vi "Read.vi"(0 "QCS in":refnum<class "QCS.lvclass">, 5 "error in (no error)":errorcluster, 6 "Force error check\nat low range":bool) -> (14 "QCS out":refnum<class "QCS.lvclass">, 15 "I0":T1 {"Current" min=0.0}, 16 "I1":T1 {"Current" min=0.0}, 17 "I2":T1 {"Current" min=0.0}, 18 "I3":T1 {"Current" min=0.0}, 19 "error out":errorcluster)   [LabVIEW 2013, in "QCS.lvclass"]
uses:
  Lib.llb/QCS.lvclass
  Lib.llb/CS Data.ctl
  Lib.llb/CS.lvclass
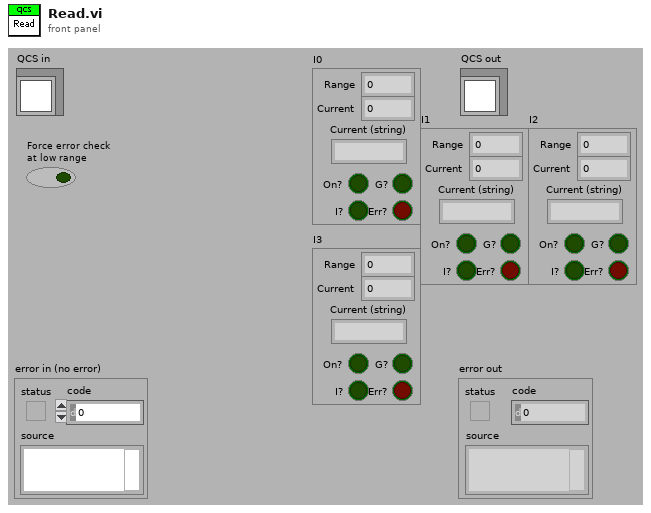
[diagram p1: front panel]
types:
  T1 = typedef "CS Data.ctl" = cluster{"Range":u8, "Current":dbl, "Current (string)":string, "On?":bool, "G?":bool, "I?":bool, "Err?":bool}
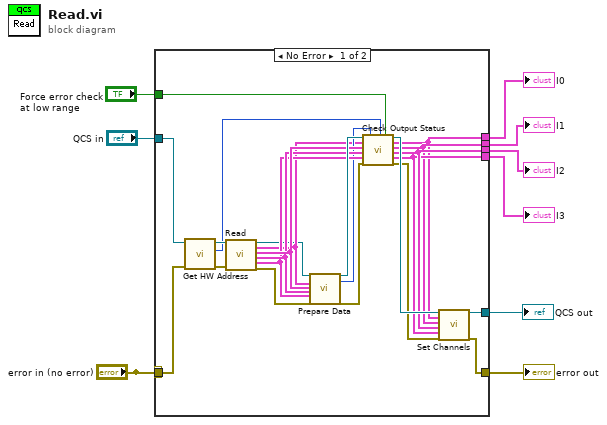
[diagram p0: block diagram]
diagram:
  n1 = case shown="No Error" "error in (no error)" {
    selector: "error in (no error)" -> [_ w33]
    tunnel: "error in (no error)" -> [w28 _]
    tunnel: [w20 w34] -> w9
    tunnel: [w10 _] -> w8
    tunnel: [w11 _] -> w7
    tunnel: [w16 _] -> w6
    tunnel: [w15 _] -> w5
    tunnel: [w18 w33] -> w4
    tunnel: "QCS in" -> [w30 w34]
    tunnel: "Force error check\nat low range" -> [w14 _]
    frame No Error {
      n2 = call-dynamic "Get HW Address.vi"("error in (no error)"=w28, "CS.lvclass in"=w30) -> ("error out"=w27:errorcluster, "HW Address"=w22:i32, "CS.lvclass out"=w29:refnum<class "QCS.lvclass">)  [unwired: 7 in]
      n3 = call-parent "Read.vi"("CS in"=w29, "error in (no error)"=w27) -> ("CS out"=w12:refnum<class "QCS.lvclass">, "I0"=w13:T1, "I1"=w25:T1, "I2"=w24:T1, "I3"=w23:T1, "error out"=w26:errorcluster)  [unwired: 12 in]
      n4 = call-dynamic "Prepare Data.vi"("CS in"=w12, "I0"=w13, "I1"=w25, "I2"=w24, "I3"=w23, "error in (no error)"=w26) -> ("Range bits"=w19:u32, "CS out"=w32:refnum<class "QCS.lvclass">, "error out"=w21:errorcluster)  [unwired: 15 in, 4 out]
      n5 = call-dynamic "Check Output Status.vi"("CS in"=w32, "I0"=w13, "I1"=w25, "I2"=w24, "I3"=w23, "error in (no error)"=w21, "Ranges"=w19, "BoardNum"=w22, "Force check"=w14) -> ("CS out"=w31:refnum<class "QCS.lvclass">, "I0 out"=w10:T1, "I1 out"=w11:T1, "I2 out"=w16:T1, "I3 out"=w15:T1, "error out"=w17:errorcluster)  [unwired: 5 in]
      n6 = call-dynamic "Set Channels.vi"("CS.lvclass in"=w31, "I0"=w10, "I1"=w11, "I2"=w16, "I3"=w15, "error in (no error)"=w17) -> ("CS.lvclass out"=w20:refnum<class "QCS.lvclass">, "error out"=w18:errorcluster)  [unwired: 12 in]
    }
    frame Error {
    }
  }
  "error out" <- w4
  "QCS out" <- w9
  "I0" <- w8
  "I1" <- w7
  "I2" <- w6
  "I3" <- w5
